vi "PAQ_ReadOneTAGdata.vi"(8 "error in (no error)":errorcluster, 10 "FetchInfo":T2, 11 "FAMM in":refnum<class "FAMM.lvclass">) -> (0 "error out":errorcluster, 2 "GraphData":T1, 3 "FAMM out":refnum<class "FAMM.lvclass">)   [LabVIEW 2014, in "FAMM.lvclass"]
doc: "Read GRAPH data from one TAG of PAQ data"
uses:
  FAMM.lvclass
  FAMM.lvclass/FAMM.ctl
  Common/controls/GlobalClassRefs.vi
  PAQ-memory.lvclass
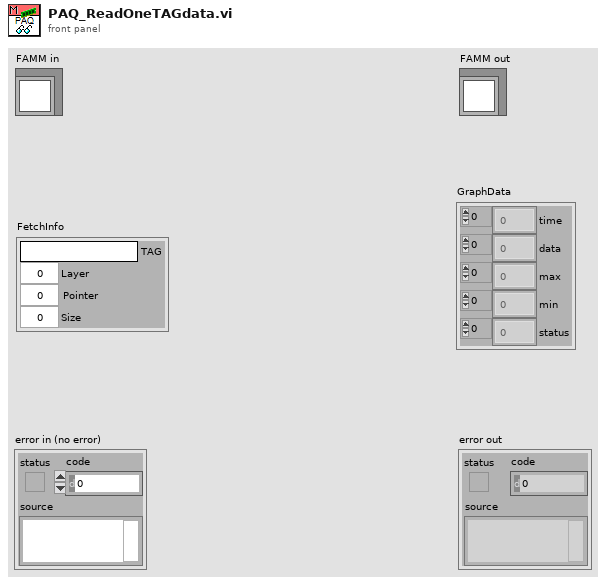
[diagram p1: front panel]
types:
  T1 = cluster{"time":dbl[], "data":dbl[], "max":dbl[], "min":dbl[], "status":u32[]}
  T2 = cluster{"TAG":string, "Layer":i32, "Pointer":i32, "Size":i32}
  T3 = cluster{"TAGindex":i32, "Location":i32, "Size":i32}
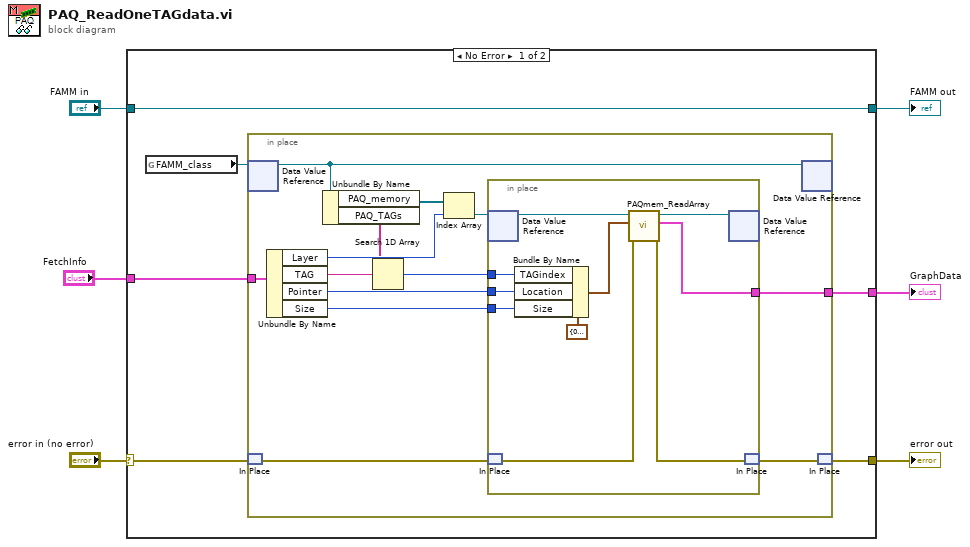
[diagram p0: block diagram]
diagram:
  n1 = case shown="No Error" "error in (no error)" {
    selector: "error in (no error)" -> [w11 w37]
    tunnel: [w10 w37] -> w5
    tunnel: [w12 w36] -> w3
    tunnel: "FAMM in" -> [w12 w36]
    tunnel: "FetchInfo" -> [w8 _]
    tunnel: [w7 _] -> w1
    frame No Error {
      n2 = global read "GlobalClassRefs.vi" "FAMM_class"() -> (w9:refnum<data-value>)
      n3 = in-place {
        in-place-border: w8 -> [w24]
        in-place-border: [w14] -> w7
        n4 = in-place-dvr #1(w9) -> (w25:refnum<class "FAMM.lvclass">)  [unwired: 1 out]
        n5 = in-place-match #2(w11) -> (w15:errorcluster)
        n6 = Unbundle By Name(w24) -> ("Layer"=w22:i32, "TAG"=w20:string, "Pointer"=w17:i32, "Size"=w16:i32)
        n7 = Unbundle By Name(w25) -> ("PAQ_memory"=w23:refnum<data-value>[], "PAQ_TAGs"=w21:string[])
        n8 = Search 1D Array(1D array=w21, element=w20) -> (index of element=w18:i32)  [unwired: 1 in]
        n9 = Index Array(array=w23, index=w22) -> (element=w19:refnum<data-value>)
        n10 = in-place {
          in-place-border: w18 -> [w31]
          in-place-border: w17 -> [w30]
          in-place-border: w16 -> [w29]
          in-place-border: [w26] -> w14
          n11 = in-place-dvr #3(w19) -> (w35:refnum<class "PAQ-memory.lvclass">)  [unwired: 1 out]
          n12 = in-place-match #4(w15) -> (w28:errorcluster)
          n13 = Bundle By Name(cluster=T3 {"TAGindex"=0, "Location"=0, "Size"=0} ("ChunkDefinition"), "TAGindex"=w31, "Location"=w30, "Size"=w29) -> (w32:T3)
          n14 = call "PAQmem_ReadArray.vi"("error in (no error)"=w28, "ChunkDefinition"=w32, "PAQ-memory in"=w35) -> ("error out"=w27:errorcluster, "GraphData"=w26:T1, "PAQ-memory out"=w34:refnum<class "PAQ-memory.lvclass">)  [unwired: 6 in]
          n15 = in-place-dvr #3(w34) -> ()  [unwired: 2 out]
          n16 = in-place-match #4(w27) -> (w13:errorcluster)
        }
        n17 = in-place-dvr #1(w25) -> ()  [unwired: 2 out]
        n18 = in-place-match #2(w13) -> (w10:errorcluster)
      }
    }
    frame Error {
    }
  }
  "error out" <- w5
  "FAMM out" <- w3
  "GraphData" <- w1
